vi "poly_control_ref_from_name_caller_single.vi"(8 "error in":errorcluster caption="Error in (no error)", 9 "control name":string, 10 "name of caller in (your caller)":string) -> (0 "error out":errorcluster, 1 "control ref":refnum<vi>, 4 "found?":bool)   [LabVIEW 2015]
uses:
  poly_ref_tools_eco_plus.vi
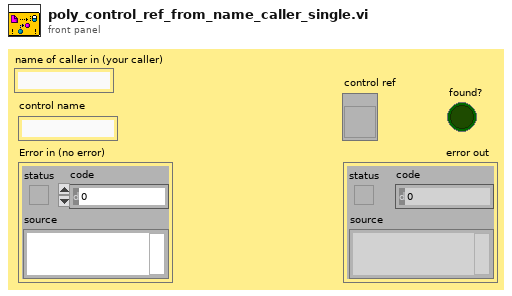
[diagram p1: front panel]
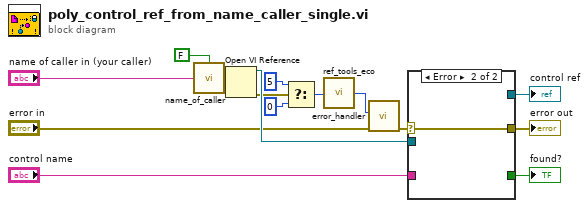
[diagram p0: block diagram]
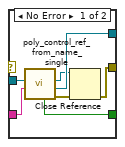
[diagram p2: hidden frame]
diagram:
  n1 = call "name_of_caller.vi"("is in inlined vi? (F)"=FALSE, "name of caller in"="name of caller in (your caller)") -> ("name of caller out"=w14:string)  [unwired: 2 in]
  n2 = Open VI Reference(vi path=w14) -> (vi reference=w10:refnum<vi>, error out=w3:errorcluster)  [unwired: 5 in]
  n3 = Select(t=5, s=w3, f=0) -> (s? t:f=w5:i32)
  n4 = call-poly "ref_tools_eco.vi"("code (w/out eco)"=w5) -> ("code (+ eco)"=w4:i32)  [unwired: 4 in]
  n5 = call "error_handler.vi"("error in (no error)"="error in", "code (0 = no error)"=w4) -> ("error out"=w1:errorcluster)  [unwired: 8 in, 1 out]
  n6 = case shown="Error" w1 {
    selector: w1 -> [_ w23]
    tunnel: [w22 w23] -> w13
    tunnel: "control name" -> [w21 _]
    tunnel: [w20 _] -> w11
    tunnel: w10 -> [w18 _]
    tunnel: [w17 _] -> w9
    frame No Error {
      n7 = call "poly_control_ref_from_name_single.vi"("control name"=w21, "vi ref"=w18) -> ("error out"=w16:errorcluster, "ctrl ref"=w20:refnum<vi>, "vi ref dup"=w19:refnum<vi>, "found?"=w17:bool)  [unwired: 6 in]
      n8 = Close Reference(reference=w19, error in (no error)=w16) -> (error out=w22:errorcluster)
    }
    frame Error {
    }
  }
  "error out" <- w13
  "control ref" <- w11
  "found?" <- w9
